vi "subVI_explodeVISAArray.vi"(7 "Array":refnum<visa-resource-name>[](array[refnum])) -> (6 "x":refnum<visa-resource-name>, 8 "y":refnum<visa-resource-name>, 10 "z":refnum<visa-resource-name>)   [LabVIEW 2013]
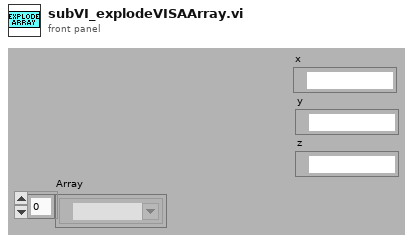
[diagram p1: front panel]
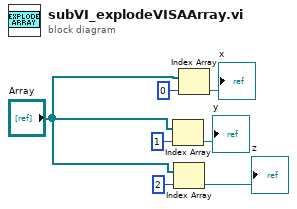
[diagram p0: block diagram]
diagram:
  n1 = Index Array(array="Array", index=1) -> (element=→"y":refnum<visa-resource-name>)
  n2 = Index Array(array="Array", index=2) -> (element=→"z":refnum<visa-resource-name>)
  n3 = Index Array(array="Array", index=0) -> (element=→"x":refnum<visa-resource-name>)
